vi "stop.vi"(8 "error in (no error)":errorcluster, 11 "ClockDL100201DAQmx in":refnum<class "ClockMT120808DAQmxSimple.lvclass">) -> (0 "error out":errorcluster, 3 "ClockDL100201DAQmx out":refnum<class "ClockMT120808DAQmxSimple.lvclass">)   [LabVIEW 2010, in "ClockMT120808DAQmxSimple.lvclass"]
doc: "Stops the generation of pulse trains. Output of pulses is stopped immediately on calling this vi even if not all the configured trains/pulses have been generated."
uses:
  ClockMT120808DAQmxSimple.lvclass
  ClockMT120808DAQmxSimple.lvclass/ClockMT120808DAQmxSimple.ctl
  GenericClock/GenericClock/GenericClock.lvclass
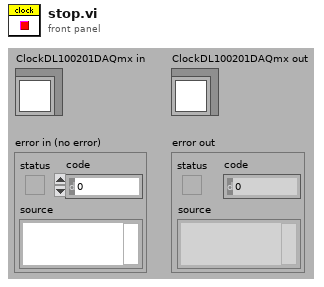
[diagram p1: front panel]
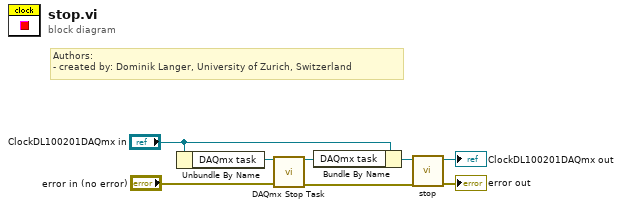
[diagram p0: block diagram]
diagram:
  # "Authors: \n- created by: Dominik Langer, University of Zurich, Switzerland"
  n1 = Unbundle By Name("ClockDL100201DAQmx in") -> ("DAQmx task"=w7:refnum<k21>)
  n2 = call <vilib>:"DAQmx Stop Task.vi"("task/channels in"=w7, "error in"="error in (no error)") -> ("task out"=w3:refnum<k21>, "error out"=w4:errorcluster)  [unwired: 12 in]
  n3 = Bundle By Name(cluster="ClockDL100201DAQmx in", "DAQmx task"=w3) -> (w1:refnum<class "ClockMT120808DAQmxSimple.lvclass">)
  n4 = call-parent "stop.vi"("error in (no error)"=w4, "GenericClock in"=w1) -> ("error out"=→"error out":errorcluster, "GenericClock out"=→"ClockDL100201DAQmx out":refnum<class "ClockMT120808DAQmxSimple.lvclass">)  [unwired: 8 in]
